vi "GenImgs.vi"(8 "error in":errorcluster, 9 "Color":u32(colorbox), 10 "Height":u32, 11 "Width":u32) -> (0 "error out":errorcluster, 3 "Imgs":picture[](array[picture]))   [LabVIEW 2012, in "Spinner.xctl"]
uses:
  Spinner.xctl
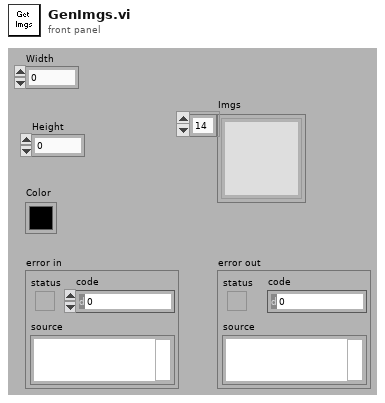
[diagram p1: front panel]
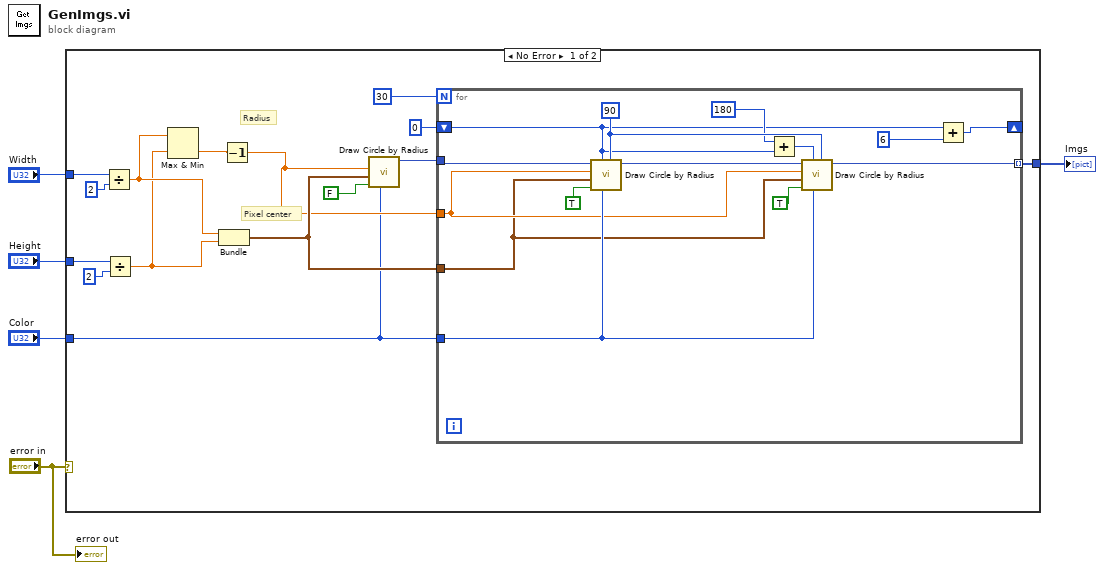
[diagram p0: block diagram]
diagram:
  n1 = case shown="No Error" "error in" {
    tunnel: "Width" -> [w12 _]
    tunnel: "Height" -> [w11 _]
    tunnel: "Color" -> [w7 _]
    tunnel: [w6 _] -> w2
    frame No Error {
      # "Radius"
      # "Pixel center"
      n2 = Divide(x=w12, y=u32 2) -> (x/y=w18:dbl)
      n3 = Divide(x=w11, y=u32 2) -> (x/y=w17:dbl)
      n4 = Max & Min(x=w18, y=w17) -> (min(x,y)=w13:dbl)  [unwired: 1 out]
      n5 = Bundle(w18, w17) -> (w10:cluster{dbl, dbl})  [unwired: 1 in]
      n6 = Decrement(x=w13) -> (x-1=w9:dbl)
      n7 = call <vilib>:"Draw Circle by Radius.vi"("color(black)"=w7, "fill?(F)"=FALSE, "pixel center"=w10, "radius"=w9) -> ("new picture"=w8:picture)  [unwired: 7 in]
      n8 = for {
        N: 30 -> [_]
        shift-right: [w21] -> _
        shift-left: 0 -> [w22]
        tunnel: w10 -> [w27]
        tunnel: w9 -> [w28]
        tunnel: w8 -> [w30]
        tunnel: w7 -> [w29]
        tunnel: [w24] -> w6 mode=indexing
        w31 = i16 90 ("arc size(360)")
        n9 = call <vilib>:"Draw Circle by Radius.vi"("arc size(360)"=w31, "color(black)"=w29, "start angle(0)"=w22, "fill?(F)"=TRUE, "pixel center"=w27, "radius"=w28, "picture"=w30) -> ("new picture"=w34:picture)  [unwired: 4 in]
        n10 = Add(x=180, y=w22) -> (x+y=w25:i32)
        n11 = call <vilib>:"Draw Circle by Radius.vi"("arc size(360)"=w31, "color(black)"=w29, "start angle(0)"=w25, "fill?(F)"=TRUE, "pixel center"=w27, "radius"=w28, "picture"=w34) -> ("new picture"=w24:picture)  [unwired: 4 in]
        n12 = Add(x=w22, y=i16 6 ("x")) -> (x+y=w21:i32)
      }
    }
    frame Error {
    }
  }
  "Imgs" <- w2
  "error out" <- "error in"
